vi "Experiment header - Update Biology info.vi"(8 "error in (no error)":errorcluster) -> (0 "error out":errorcluster)   [LabVIEW 2017]
uses:
  Typedefs/Header file interface module functions enum.ctl
  Typedefs/Header file sections.ctl
  Typedefs/Header parameters cluster-ALL.ctl
  Typedefs/Header subclusters/Header params -Login.ctl
  Typedefs/Header subclusters/Header params-Global Parameters.ctl
  Misc/Experiment Type.ctl
  Typedefs/Header subclusters/Header params-Imaging Modes.ctl
  Typedefs/Header subclusters/Header params-Time Series.ctl
  Typedefs/Header subclusters/Header params-Basic image meta data.ctl
  Typedefs/Frame Size.ctl
  Typedefs/Header subclusters/Header params-Motor Z-stack.ctl
  Typedefs/Header subclusters/Header params-AOL Z-stack.ctl
  Typedefs/Header subclusters/Header params-Functional Imaging.ctl
  Typedefs/Functional Mode.ctl
  Typedefs/AOL modes.ctl
  Typedefs/Plane Mode.ctl
  Typedefs/Header subclusters/Header params-Calibration Setup.ctl
  Typedefs/Header subclusters/Header params-statistics.ctl
  Misc/Biology Information.ctl
  Global Variables/gl_UI Ctrl Refs.vi
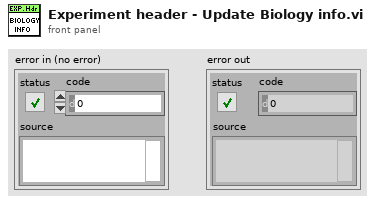
[diagram p1: front panel]
types:
  T1 = typedef "Header parameters cluster-ALL.ctl" = cluster{"LOGIN":T2, "GLOBAL PARAMETERS":T3, "IMAGING MODES":T5, "TIME SERIES":T6, "MOTOR Z-STACK ":T9, "AOL Z-STACK":T10, "FUNCTIONAL IMAGING":T11, "VOLUME IMAGING":T11, "CALIBRATION":T15, "STATISTICS":T16, "BIOLOGY INFORMATION":T17}
  T2 = typedef "Header params -Login.ctl" = cluster{"User":string, "Profile":string, "Software Version":string, "Experiment Date Time":timestamp}
  T3 = typedef "Header params-Global Parameters.ctl" = cluster{"MicroscopeID":string, "Microscope Type":string, "Objective":string, "Field of View (um)":dbl, "Fill time (us)":dbl, "Experiment Type":T4, "Stimuli Trigger":bool, "Speed Logging":bool}
  T4 = typedef "Experiment Type.ctl" = enum16{"In vivo", "In vitro", "Testing", "Calibration", "Other"}
  T5 = typedef "Header params-Imaging Modes.ctl" = cluster{"Time Series":bool, "Motor Zstack":bool, "AOL Zstack":bool, "Functional Imaging":bool, "Volume Imaging":bool}
  T6 = typedef "Header params-Time Series.ctl" = cluster{"Basic Image meta data":T7, "AOL z":dbl}
  T7 = typedef "Header params-Basic image meta data.ctl" = cluster{"Wavelength (nm)":dbl, "# averaged frames":dbl, "laser power (%)":dbl, "Pockels":dbl, "pixel dwell time (us)":dbl, "pmt 1":dbl, "pmt 2":dbl, "back apperture":dbl, "zoom":dbl, "field of view":dbl, "Frame Size":T8, "AOL x centre":dbl, "AOL y centre":dbl, "Stage x position":dbl, "Stage y position":dbl, "Stage z position":dbl}
  T8 = typedef "Frame Size.ctl" = u16
  T9 = typedef "Header params-Motor Z-stack.ctl" = cluster{"Hdr Basic Image meta data":T7, "Z Start":dbl, "Z Stop":dbl, "No of Planes":i32}
  T10 = typedef "Header params-AOL Z-stack.ctl" = cluster{"Hdr Basic Image meta data":T7, "Z Start":dbl, "Z Stop":dbl, "No of Planes":i32}
  T11 = typedef "Header params-Functional Imaging.ctl" = cluster{"Functional Mode":T12, "Pockels Modulation":bool, "Number of pois":dbl, "Number of miniscans":dbl, "Number of cycles":dbl, "Number of trials":dbl, "Miniscan dwell time per pixel (us)":dbl, "Number of pixels in miniscan":dbl, "poi dwell time":dbl, "Rectangle ROI length":dbl, "Rectangle ROI height":dbl, "AOL Mode":T13, "Plane Mode":T14, "video length (sec)":dbl, "Frame rate (fps)":dbl, "Stimuli Timing (usec)":dbl, "Acquisition Length":dbl, "Basic Image meta data":T7, "Z Start (um)":dbl, "Z Stop (um)":dbl}
  T12 = typedef "Functional Mode.ctl" = enum16{"Point", "Line", "Patch", "Plane", "Volume"}
  T13 = typedef "AOL modes.ctl" = enum16{"Raster", "Structural", "Pointing", "Mini Scan", "Alignment"}
  T14 = typedef "Plane Mode.ctl" = u16
  T15 = typedef "Header params-Calibration Setup.ctl" = cluster{"Pockels Calibration File":path, "Calibration_ini file":path, "Setup_ini file":path}
  T16 = typedef "Header params-statistics.ctl" = cluster{"Z-stack duration (sec)":dbl, "Number of acquired data-points":dbl, "Acquisition time (ms)":dbl, "Number of acquired frames":dbl, "Intertrial times":dbl[]}
  T17 = typedef "Biology Information.ctl" = cluster{"Animal Code or Name":string, "Animal DoB":string, "Animal Age":string, "Animal Sex":string, "Animal Weight":string, "Date of Injection":string, "Date of Implant":string, "Site of Injection":string, "Animal Ear Notch":string, "AAV constructs":string, "Genetic background":string, "Optical reporter":string, "Region of brain imaged":string, "Other \ncomments":string}
  T18 = typedef "Header file sections.ctl" = enum16{"ALL SECTIONS", "LOGIN", "GLOBAL PARAMETERS", "IMAGING MODES", "TIME SERIES", "MOTOR Z-STACK", "AOL Z-STACK", "FUNCTIONAL IMAGING", "VOLUME IMAGING", "CALIBRATION", "STATISTICS", "BIOLOGY INFORMATION"}
  T19 = typedef "Header file interface module functions enum.ctl" = enum16{"Load experiment header file", "Save experiment header file", "Clear stored values", "Read stored values", "Update specific value in memory", "Update values in memory"}
  T20 = typedef "UI ctrl refs cluster.ctl" = cluster{"Top level VI path":path, "Top level VI ref":refnum<vi>, "User menu ref":refnum<k9>, "Sub Panel control":refnum<vi>, "Imaging Param Tab":refnum<vi>, "Occurrence-Start drivers":refnum<k4>, "Occurrence-Speed logging initialised":refnum<k4>, "Occurrence-XYZ stage initialised":refnum<k4>, "Exit button":refnum<vi>, "Status ind":refnum<vi>, "Set as origin":refnum<vi>, "Speed Logging":refnum<vi>, "Time Lapse":refnum<vi>, "Live Imaging":refnum<vi>, "AOL Z Stack":refnum<vi>, "Motor Z Stack":refnum<vi>, "Funct Acq button":refnum<vi>, "Hard Shutter":refnum<vi>, "Virtual Shutter":refnum<vi>, "Laser Power":refnum<vi>, "AOL Mode":refnum<vi>, "Frame Size":refnum<vi>, "Field of View":refnum<vi>, "Dwell Time":refnum<vi>, "Zoom":refnum<vi>, "AOL Z":refnum<vi>, "Objective":refnum<vi>, "Axis":refnum<vi>, "Paths & Names":refnum<vi>, "Experiment folder path (ind.)":refnum<vi>, "Last State (Ind.)":refnum<vi>, "Averages":refnum<vi>, "Angle (degrees)":refnum<vi>, "X centre":refnum<vi>, "Y centre":refnum<vi>, "Plane Mode":refnum<vi>, "# Planes":refnum<vi>, "Z Start":refnum<vi>, "Z Stop":refnum<vi>, "Z Step":refnum<vi>, "PMT 1":refnum<vi>, "PMT 2":refnum<vi>, "Stage XYZ Position":refnum<vi>, "Pockels@Z Start":refnum<vi>, "Pockels@Z Stop":refnum<vi>, "Obtain Z Start":refnum<vi>, "Obtain Z Stop":refnum<vi>, "Live stim.trig.period":refnum<vi>, "Live stim.trig.enable":refnum<vi>, "XY Stage Move":refnum<vi>, "Funct. Acq. Pockels Modulation":refnum<vi>, "Enable Video Recording":refnum<vi>, "Video Record-Live Imaging":refnum<vi>, "Video Record-Funct acq":refnum<vi>, "AOL Z-stack Chirps Ready (ind)":refnum<vi>, "Center freq ind (nm)":refnum<vi>, "Pickup mode (ind)":refnum<vi>, "Logging queue (ind)":refnum<vi>, "Back aperture power (ind.)":refnum<vi>, "Power after objective (ind.)":refnum<vi>, "Switch user":refnum<vi>, "Ls1 Conn. Status":refnum<vi>, "Ls1Tuning Status":refnum<vi>, "Ls1 Faults":refnum<vi>, "Ls1 Connection":refnum<vi>, "Ls1 Mode":refnum<vi>, "Ls1 POWER [mW]":refnum<vi>, "Ls1Shutter":refnum<vi>, "Ls1 Wavelength":refnum<vi>, "Ls1 Note":refnum<vi>, "Ls1 Confirm Wav":refnum<vi>, "Ls1 PreChrp Prism1":refnum<vi>, "Ls1 PreChrp Prism2":refnum<vi>, "Ls1 wav top Ind":refnum<vi>, "Ls1 power top Ind":refnum<vi>, "Ls1 Pump peak Hold":refnum<vi>, "Ls1 Status Ind":refnum<vi>, "Ls1 wav cancel":refnum<vi>, "Experiment Type":refnum<vi>, "Biology Information":refnum<vi>}
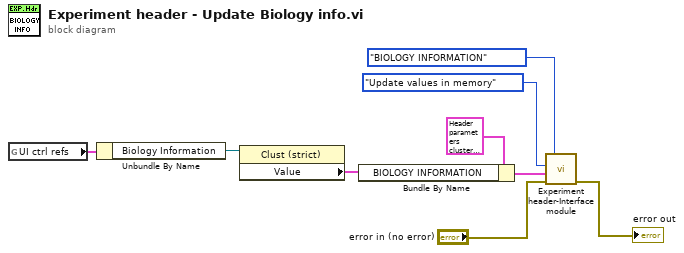
[diagram p0: block diagram]
diagram:
  n1 = global read "gl_UI Ctrl Refs.vi" "UI ctrl refs"() -> (w5:T20)
  n2 = Unbundle By Name(w5) -> ("Biology Information"=w4:refnum<vi>)
  n3 = property class="Clust (strict)"(reference=w4) -> ("Value"=w2:T17)  [unwired: 1 in, 2 out]
  n4 = Bundle By Name(cluster=T1 {"LOGIN"={"User"="Olympus  20X", "Profile"="", "Software Version"="", "Experiment Date Time"=timestamp(0 s since 1904-01-01)}, "GLOBAL PARAMETERS"={"MicroscopeID"="", "Microscope Type"="", "Objective"="", "Field of View (um)"=0.0, "Fill time (us)"=0.0, "Experiment Type"=enum."In vivo", "Stimuli Trigger"=FALSE, "Speed Logging"=FALSE}, "IMAGING MODES"={"Time Series"=FALSE, "Motor Zstack"=FALSE, "AOL Zstack"=FALSE, "Functional Imaging"=FALSE, "Volume Imaging"=FALSE}, "TIME SERIES"={"Basic Image meta data"={"Wavelength (nm)"=0.0, "# averaged frames"=0.0, "laser power (%)"=0.0, "Pockels"=0.0, "pixel dwell time (us)"=0.0, "pmt 1"=0.0, "pmt 2"=0.0, "back apperture"=0.0, "zoom"=0.0, "field of view"=0.0, "Frame Size"=0, "AOL x centre"=0.0, "AOL y centre"=0.0, "Stage x position"=0.0, "Stage y position"=0.0, "Stage z position"=0.0}, "AOL z"=0.0}, "MOTOR Z-STACK "={"Hdr Basic Image meta data"={"Wavelength (nm)"=0.0, "# averaged frames"=0.0, "laser power (%)"=0.0, "Pockels"=0.0, "pixel dwell time (us)"=0.0, "pmt 1"=0.0, "pmt 2"=0.0, "back apperture"=0.0, "zoom"=0.0, "field of view"=0.0, "Frame Size"=0, "AOL x centre"=0.0, "AOL y centre"=0.0, "Stage x position"=0.0, "Stage y position"=0.0, "Stage z position"=0.0}, "Z Start"=0.0, "Z Stop"=0.0, "No of Planes"=0}, "AOL Z-STACK"={"Hdr Basic Image meta data"={"Wavelength (nm)"=0.0, "# averaged frames"=0.0, "laser power (%)"=0.0, "Pockels"=0.0, "pixel dwell time (us)"=0.0, "pmt 1"=0.0, "pmt 2"=0.0, "back apperture"=0.0, "zoom"=0.0, "field of view"=0.0, "Frame Size"=0, "AOL x centre"=0.0, "AOL y centre"=0.0, "Stage x position"=0.0, "Stage y position"=0.0, "Stage z position"=0.0}, "Z Start"=0.0, "Z Stop"=0.0, "No of Planes"=0}, "FUNCTIONAL IMAGING"={"Functional Mode"=enum."Point", "Pockels Modulation"=FALSE, "Number of pois"=0.0, "Number of miniscans"=0.0, "Number of cycles"=0.0, "Number of trials"=0.0, "Miniscan dwell time per pixel (us)"=0.0, "Number of pixels in miniscan"=0.0, "poi dwell time"=0.0, "Rectangle ROI length"=0.0, "Rectangle ROI height"=0.0, "AOL Mode"=enum."Raster", "Plane Mode"=0, "video length (sec)"=0.0, "Frame rate (fps)"=0.0, "Stimuli Timing (usec)"=0.0, "Acquisition Length"=0.0, "Basic Image meta data"={"Wavelength (nm)"=0.0, "# averaged frames"=0.0, "laser power (%)"=0.0, "Pockels"=0.0, "pixel dwell time (us)"=0.0, "pmt 1"=0.0, "pmt 2"=0.0, "back apperture"=0.0, "zoom"=0.0, "field of view"=0.0, "Frame Size"=0, "AOL x centre"=0.0, "AOL y centre"=0.0, "Stage x position"=0.0, "Stage y position"=0.0, "Stage z position"=0.0}, "Z Start (um)"=0.0, "Z Stop (um)"=0.0}, "VOLUME IMAGING"={"Functional Mode"=enum."Point", "Pockels Modulation"=FALSE, "Number of pois"=0.0, "Number of miniscans"=0.0, "Number of cycles"=0.0, "Number of trials"=0.0, "Miniscan dwell time per pixel (us)"=0.0, "Number of pixels in miniscan"=0.0, "poi dwell time"=0.0, "Rectangle ROI length"=0.0, "Rectangle ROI height"=0.0, "AOL Mode"=enum."Raster", "Plane Mode"=0, "video length (sec)"=0.0, "Frame rate (fps)"=0.0, "Stimuli Timing (usec)"=0.0, "Acquisition Length"=0.0, "Basic Image meta data"={"Wavelength (nm)"=0.0, "# averaged frames"=0.0, "laser power (%)"=0.0, "Pockels"=0.0, "pixel dwell time (us)"=0.0, "pmt 1"=0.0, "pmt 2"=0.0, "back apperture"=0.0, "zoom"=0.0, "field of view"=0.0, "Frame Size"=0, "AOL x centre"=0.0, "AOL y centre"=0.0, "Stage x position"=0.0, "Stage y position"=0.0, "Stage z position"=0.0}, "Z Start (um)"=0.0, "Z Stop (um)"=0.0}, "CALIBRATION"={"Pockels Calibration File"=path "", "Calibration_ini file"=path "", "Setup_ini file"=path ""}, "STATISTICS"={"Z-stack duration (sec)"=0.0, "Number of acquired data-points"=0.0, "Acquisition time (ms)"=0.0, "Number of acquired frames"=0.0, "Intertrial times"=[]}, "BIOLOGY INFORMATION"={"Animal Code or Name"="", "Animal DoB"="", "Animal Age"="", "Animal Sex"="", "Animal Weight"="", "Date of Injection"="", "Date of Implant"="", "Site of Injection"="", "Animal Ear Notch"="", "AAV constructs"="", "Genetic background"="", "Optical reporter"="", "Region of brain imaged"="", "Other \ncomments"=""}} ("All header parameters in"), "BIOLOGY INFORMATION"=w2) -> (w1:T1)
  n5 = call "Experiment header-Interface module.vi"("Header file sections"=Header_file_sections."BIOLOGY INFORMATION", "error in (no error)"="error in (no error)", "All header parameters in"=w1, "Function"=Header_file_interface_module_functions_enum."Update values in memory") -> ("error out"=→"error out":errorcluster)  [unwired: 6 in, 1 out]
